vi "calculate_span.vi"(7 "Sweep in":T2={"DorG_0"="", "Vvar_0_start"=0.0, "Vvar_0_step"=0.0, "Vvar_0_Stop"=0.0, "Vvar_1_start "=0.0, "Drain Current Compliance"=1e-06, "Gate Current Compliance 0"=1e-06, "Vvar_0_holdtime"=0.0, "Vvar-0_delaytime"=0.0, "IntPts_0"=100.0, "Set Swe_0_Mode"="", "Sweep Spacing_0"=""}, 11 "V_points":dbl) -> (0 "Gate Point number Checker":string, 1 "Gate Potential_checker":string, 3 "V Step":dbl, 6 "Sweep out":T1={"DorG"="", "Vvar_start"=0.0, "Vvar_step"=0.0, "Vvar_Stop"=0.0, "V_const "=0.0, "Drain Current Compliance"=1e-06, "Gate Current Compliance"=1e-06, "Vvar_holdtime"=0.0, "Vvar_delaytime"=0.0, "IntPts"=100.0, "Set Swe_Mode"="", "Sweep Spacing"=""})   [LabVIEW 2021]
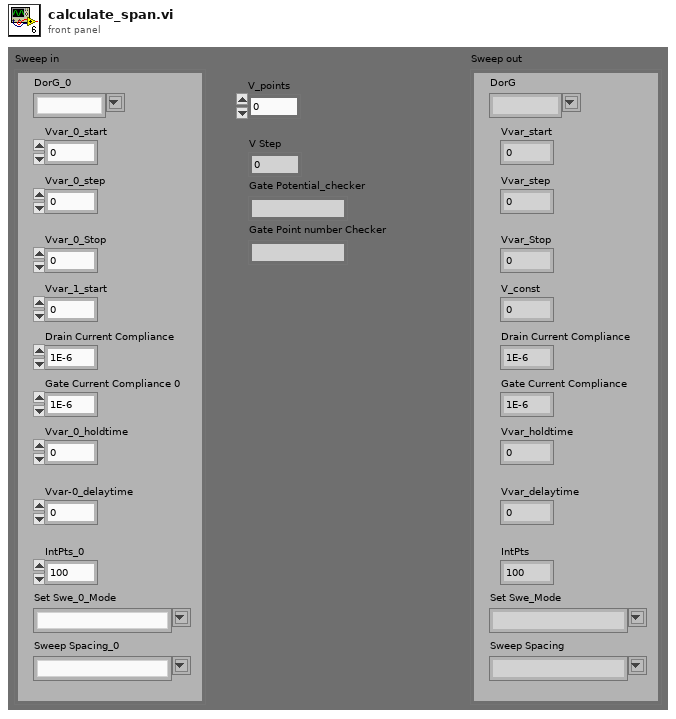
[diagram p1: front panel]
types:
  T1 = cluster{"DorG":string, "Vvar_start":dbl, "Vvar_step":dbl, "Vvar_Stop":dbl, "V_const ":dbl, "Drain Current Compliance":dbl, "Gate Current Compliance":dbl, "Vvar_holdtime":dbl, "Vvar_delaytime":dbl, "IntPts":dbl, "Set Swe_Mode":string, "Sweep Spacing":string}
  T2 = cluster{"DorG_0":string, "Vvar_0_start":dbl, "Vvar_0_step":dbl, "Vvar_0_Stop":dbl, "Vvar_1_start ":dbl, "Drain Current Compliance":dbl, "Gate Current Compliance 0":dbl, "Vvar_0_holdtime":dbl, "Vvar-0_delaytime":dbl, "IntPts_0":dbl, "Set Swe_0_Mode":string, "Sweep Spacing_0":string}
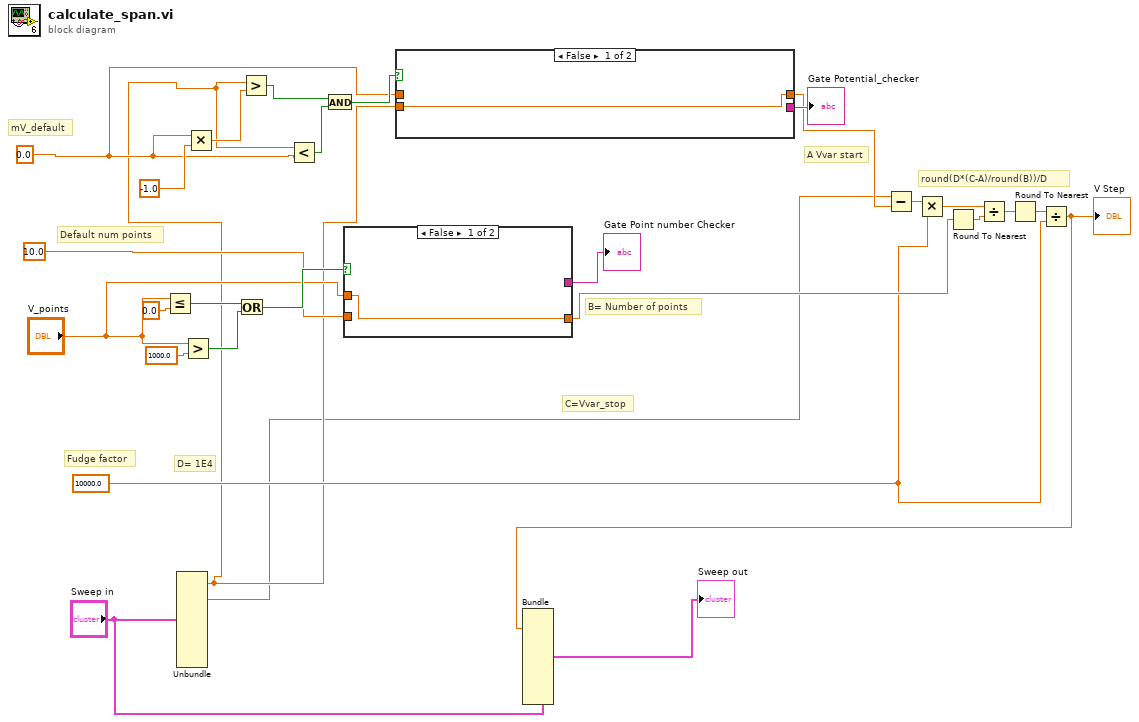
[diagram p0: block diagram]
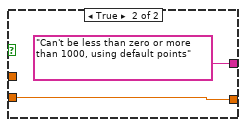
[diagram p2: hidden frame]
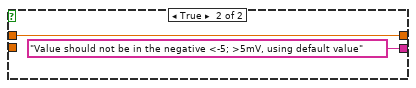
[diagram p3: hidden frame]
diagram:
  w7 = 0.0 ("Default mV start")
  w8 = 10000.0
  # "Default num points"
  # "mV_default"
  # "round(D*(C-A)/round(B))/D"
  # "Fudge factor"
  # "D= 1E4"
  # "B= Number of points"
  # "C=Vvar_stop"
  # "A Vvar start"
  n1 = Less Or Equal?(x="V_points", y=0.0) -> (x <= y?=w19:bool)
  n2 = Unbundle("Sweep in") -> ("Vvar_0_start"=w5:dbl, "Vvar_0_Stop"=w4:dbl)  [unwired: 10 out]
  n3 = Greater?(x="V_points", y=1000.0) -> (0:w18:bool)
  n4 = Multiply(x=w7, y=-1.0) -> (x*y=w27:dbl)
  n5 = Or(x=w19, y=w18) -> (x .or. y?=w17:bool)
  n6 = Greater?(x=w5, y=w27) -> (0:w26:bool)
  n7 = Less?(x=w5, y=w7) -> (x < y?=w25:bool)
  n8 = And(x=w26, y=w25) -> (x .and. y?=w24:bool)
  n9 = case shown="False" w17 {
    tunnel: 10.0 ("Default_Number of points") -> [_ w31]
    tunnel: [w29 w31] -> w14
    tunnel: "V_points" -> [w29 _]
    tunnel: [_ "Can't be less than zero or more than 1000, using default points"] -> w15
    frame False {
    }
    frame True {
    }
  }
  "Gate Point number Checker" <- w15
  n10 = case shown="False" w24 {
    tunnel: [_ "Value should not be in the negative <-5; >5mV, using default value"] -> w23
    tunnel: w7 -> [_ w33]
    tunnel: [w32 w33] -> w22
    tunnel: w5 -> [w32 _]
    frame False {
    }
    frame True {
    }
  }
  "Gate Potential_checker" <- w23
  n11 = Subtract(x=w4, y=w22) -> (x-y=w13:dbl)
  n12 = Multiply(x=w13, y=w8) -> (x*y=w12:dbl)
  n13 = Round To Nearest(number=w14) -> (nearest integer value=w11:dbl)
  n14 = Divide(x=w12, y=w11) -> (x/y=w10:dbl)
  n15 = Round To Nearest(number=w10) -> (nearest integer value=w9:dbl)
  n16 = Divide(x=w9, y=w8) -> (x/y=w2:dbl)
  "V Step" <- w2
  n17 = Bundle(cluster="Sweep in", "Vvar_0_step"=w2) -> (→"Sweep out":T2)  [unwired: 11 in]
